vi "armff-battery-sim-exec.vi"(10 "Nominal Battery Voltge":dbl, 11 "Current":dbl) -> (3 "Actual Battery Voltage":dbl)   [LabVIEW 2019]
uses:
  <vilib>/Rock Robotics/WPI/ThirdParty/JAS_Junk/TrajLib/Trajectory_Library.lvlib
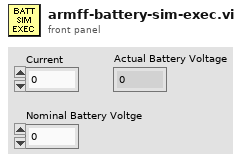
[diagram p1: front panel]
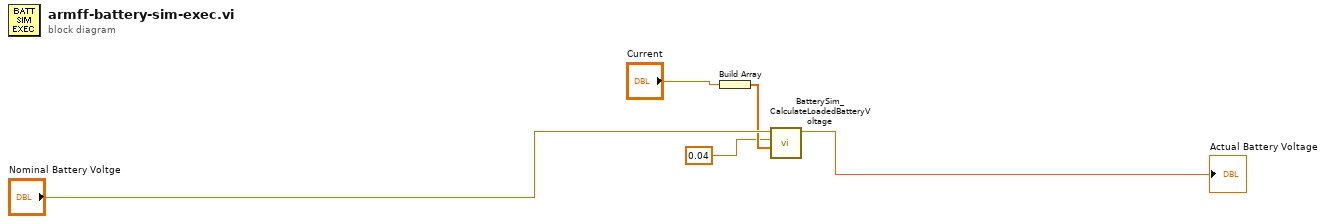
[diagram p0: block diagram]
diagram:
  n1 = Build Array("Current") -> (w2:dbl[])
  n2 = call <vilib>:"BatterySim_CalculateLoadedBatteryVoltage.vi"("Currents"=w2, "Resistance_Ohms"=0.04, "NominalVoltage"="Nominal Battery Voltge") -> ("Voltage"=→"Actual Battery Voltage":dbl)  [unwired: 8 in]
